vi "Exp no 11 Signal Generation Using LABVIEW.vi"() -> ()   [LabVIEW 2010]
uses:
  <vilib>/measure/NI_MABase.lvlib
panel:
  in  "Signal Type":T1(ring)
  out "Waveform Graph":waveform(dbl)(graph)
  in  "Stop":bool
  in  "Frequency":u16(knob) scale=0.0..10.0
  in  "Amplitude":u16(knob) scale=0.0..10.0
  # "SIGNAL GENERATION USING LABVIEW"
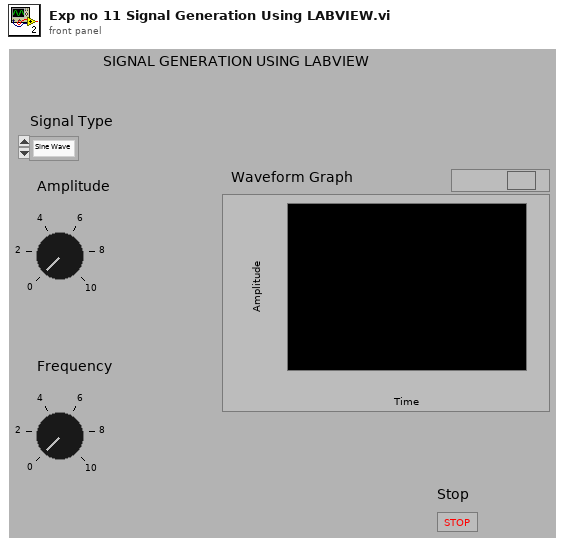
[diagram p1: front panel]
types:
  T1 = enum16{"Sine Wave", "Triangle Wave", "Square Wave", "Sawtooth Wave"}
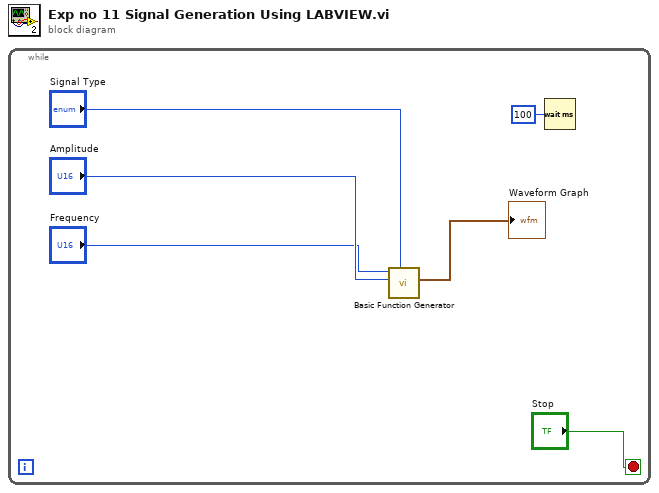
[diagram p0: block diagram]
diagram:
  n1 = while {
    stop <- "Stop" stop-if-true
    n2 = call <vilib>:"Basic Function Generator.vi"("signal type"="Signal Type", "amplitude"="Amplitude", "frequency"="Frequency") -> ("signal out"=→"Waveform Graph":waveform(dbl))  [unwired: 6 in, 2 out]
    n3 = Wait (ms)(milliseconds to wait=u32 100) -> ()  [unwired: 1 out]
  }
